vi "CFPI.vi"() -> ()   [LabVIEW 2014]
uses:
  <vilib>/Utility/file.llb/Write To Spreadsheet File (DBL).vi
panel:
  out "Elapsed time":dbl
  in  "Sin intervals":u32=40 caption="Sin" min=1 step=1
  in  "stop":bool
  in  "Matlab / Excel":bool
  in  "D intervals":u32=40 caption="D" min=1 step=1
  in  "Speed":u32=1 min=1 step=1
  in  "Scaled Time simulation":bool
  in  "Automatic D":bool caption="Automatic D values"
  in  "Write to file":bool
  in  "Initial conditions":bool
  in  "D_max":dbl=0.25 min=0.0 step=0.001 format="%#.5f"
  in  "D_min":dbl=0.01 min=0.0 step=0.001 format="%#.5f"
  in  "Do":dbl=40.0 caption="Sin_max" min=0.0
  in  "Od":dbl caption="Sin_min" min=0.0
  in  "czas pomiaru":dbl=400.0 caption="Measurement time"
  in  "czas stabilizacji":dbl=600.0 caption="Response formation time"
  out "D":dbl format="%.3f"
  out "X Chart":dbl(graph) caption="P Chart 2"
  out "P Chart":dbl(graph)
  in  "Tab Control":T1(tab)
  out "XY Graph 1":cluster{dbl[], dbl[]}[](graph)
  out "XY Graph 2":cluster{dbl[], dbl[]}[](graph)
  out "XY Graph 3":cluster{dbl[], dbl[]}[](graph)
  out "XY Graph 4":cluster{dbl[], dbl[]}[](graph)
  out "XY Graph 5":cluster{dbl[], dbl[]}[](graph)
  in  "tau":dbl=23.0 caption="delay"
  in  "S(0)":dbl
  in  "X(0)":dbl=1.0
  in  "P(0)":dbl
  in  "NIS":u32=10
  in  "Dt":dbl=0.1
  in  "Yp":dbl=3.68
  in  "Y":dbl=0.108
  in  "Ki":dbl=3.069
  in  "um":dbl=0.282 caption="m_m"
  in  "Ks":dbl=0.025
  in  "D5":dbl=0.25 caption="5" format="%#.5f"
  in  "D4":dbl=0.15 caption="4" format="%#.5f"
  in  "D3":dbl=0.1 caption="3" format="%#.5f"
  in  "D2":dbl=0.05 caption="2" format="%#.5f"
  in  "D1":dbl=0.01 caption="1" format="%#.5f"
  out "Sin":dbl format="%.3f"
  out "Substrate":dbl format="%.3f"
  out "Biomass":dbl format="%.3f"
  out "Product":dbl format="%.3f"
  out "Tank":cluster{dbl, dbl, dbl}(slide) scale=0.0..40.0
  # "Number of intervals"
  # "[s]"
  # "[h]"
  # "[h]"
  # "[g/L]"
  # "[g/L]"
  # "[1/h]"
  # "[1/h]"
  # "[1/h]"
  # "Parameters"
  # "Initial conditions"
  # "[1/h]"
  # "[g/L]"
  # "[g/L]"
  # "[g/L]"
  # "[g/L]"
  # "[g/L]"
  # "[g/g]"
  # "Simulation resolution"
  # "[g/g]"
  # "[h]"
  # "[h]"
  # "Manual D [1/h]"
  # "[g/L]"
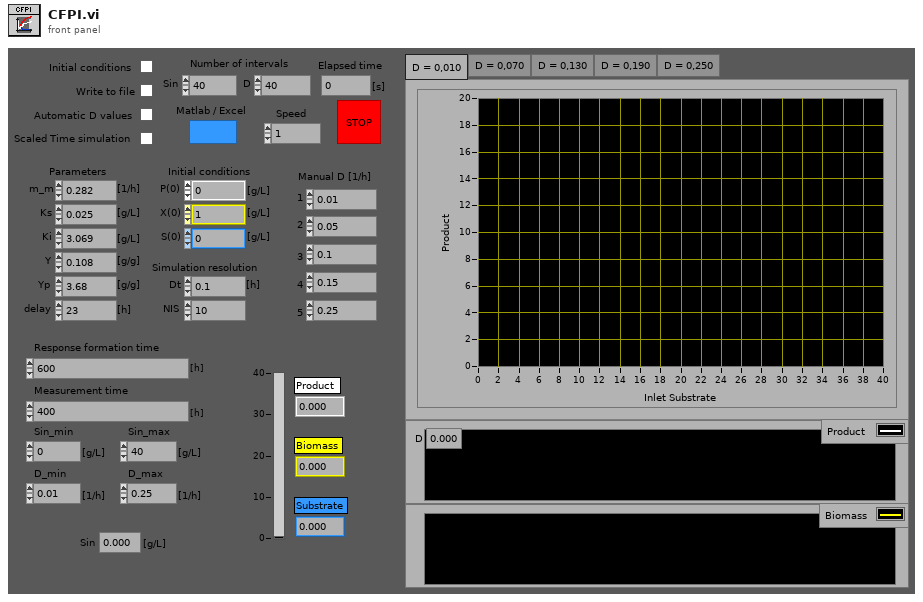
[diagram p1: front panel]
types:
  T1 = enum32{"Page 1", "Page 2", "Page 3", "Page 4", "Page 5"}
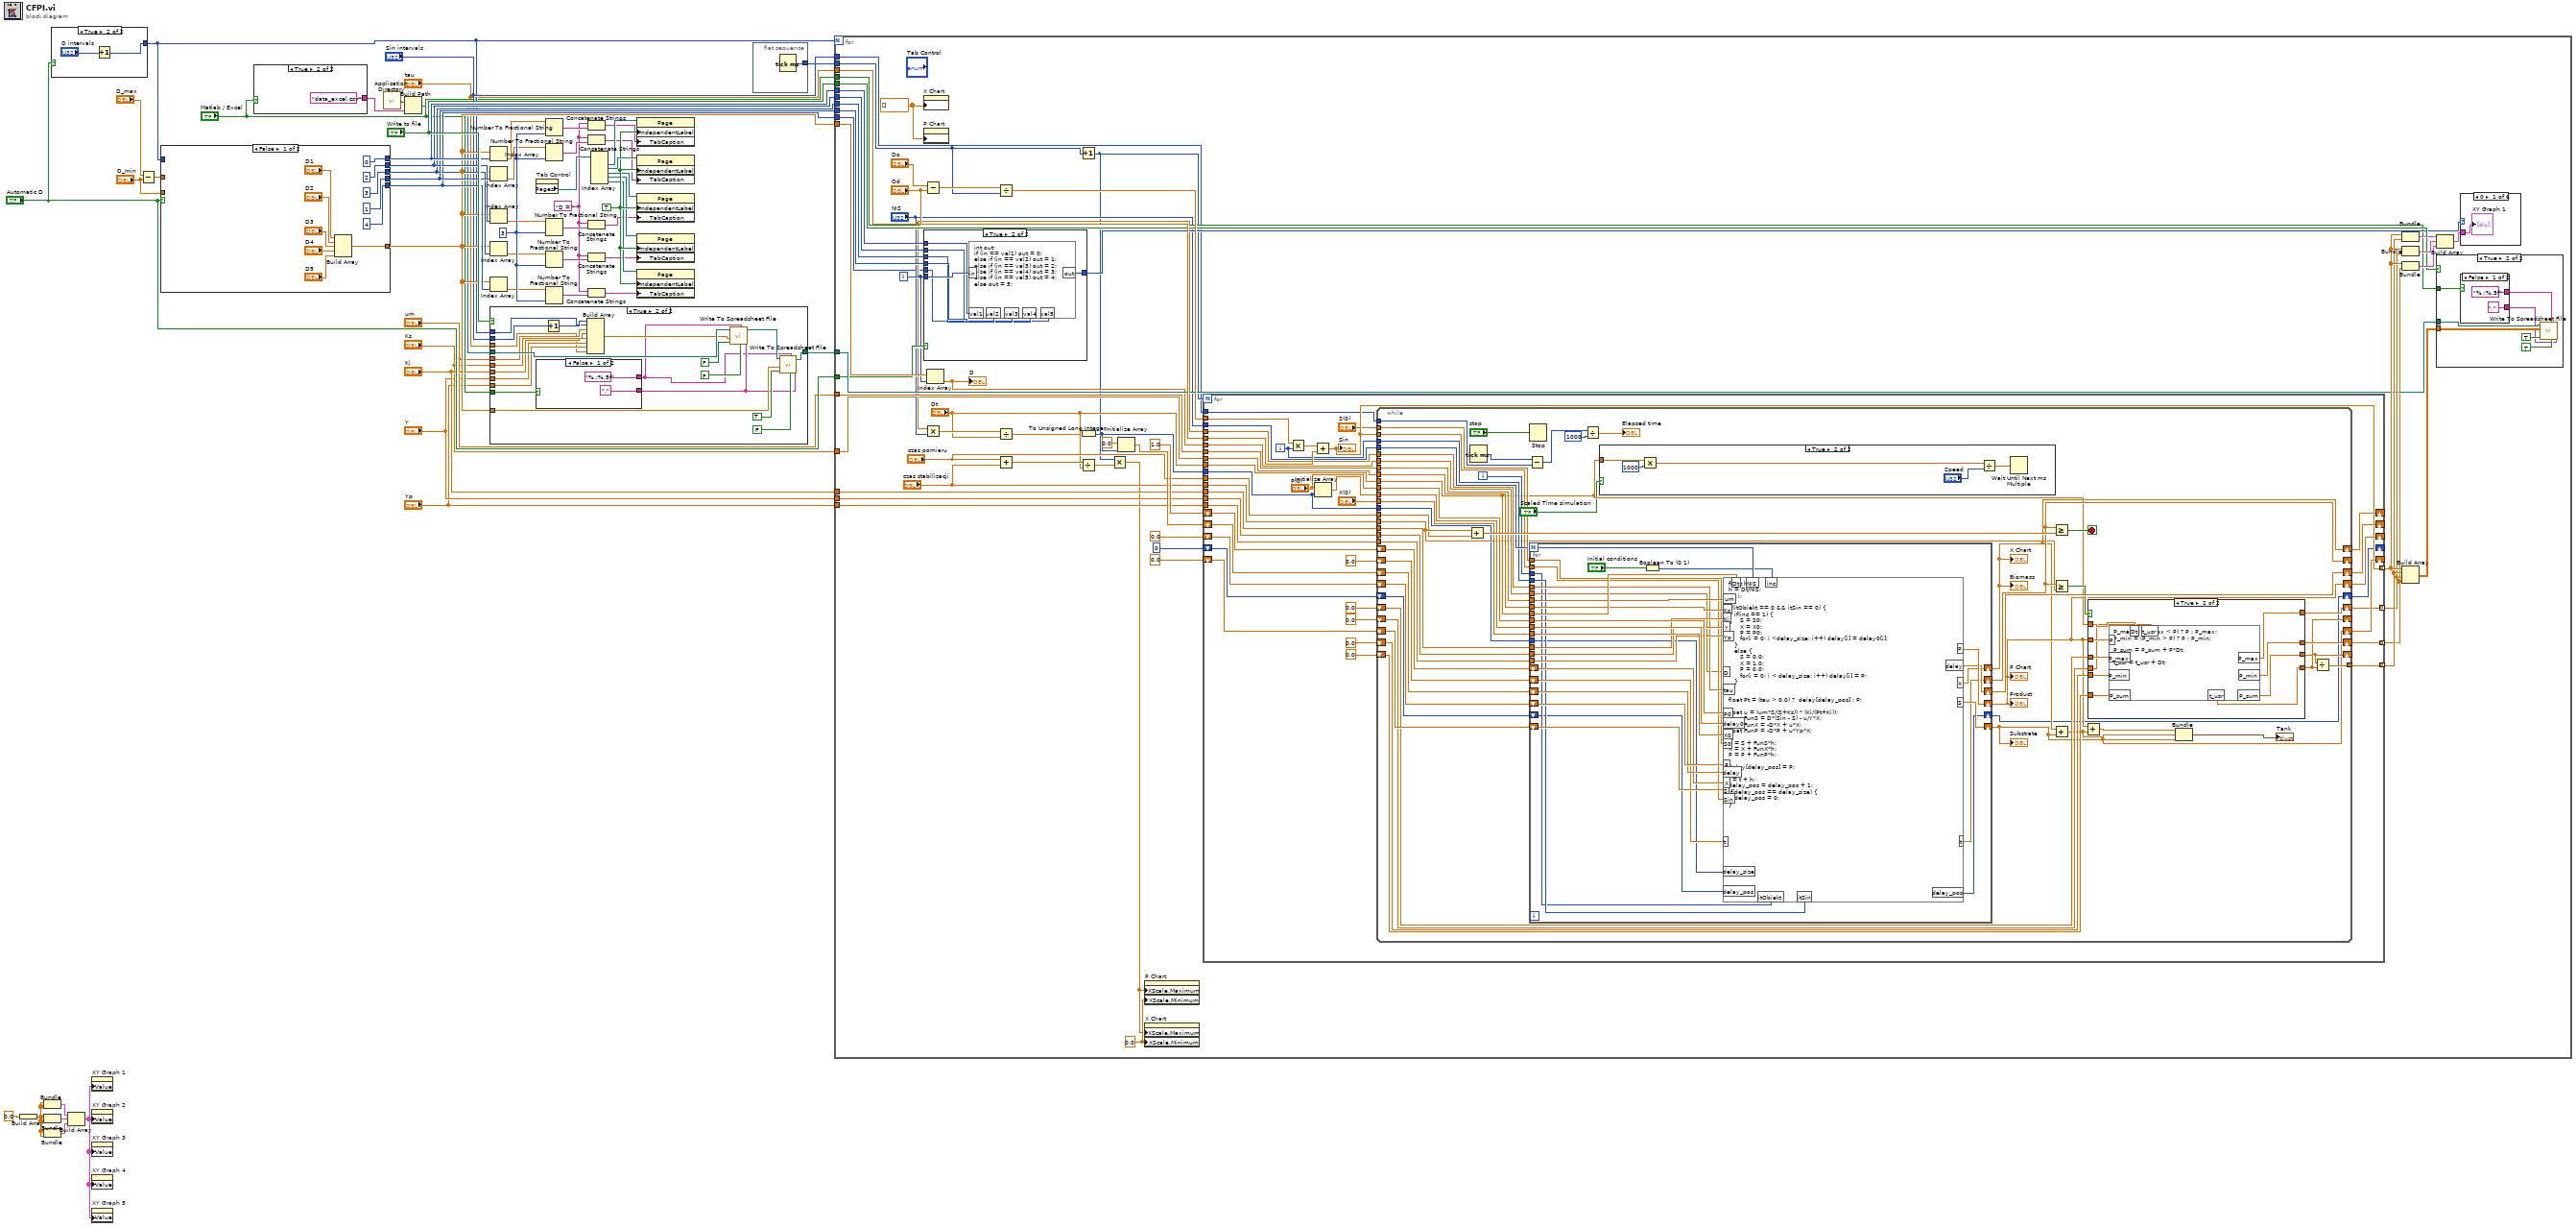
[diagram p0: block diagram]
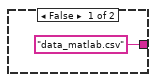
[diagram p2: hidden frame]
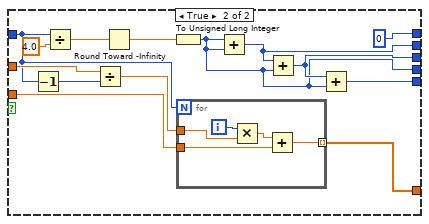
[diagram p3: hidden frame]
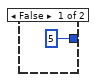
[diagram p4: hidden frame]
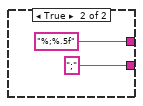
[diagram p6: hidden frame]
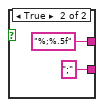
[diagram p9: hidden frame]
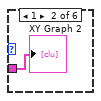
[diagram p10: hidden frame]
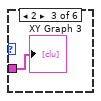
[diagram p11: hidden frame]
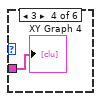
[diagram p12: hidden frame]
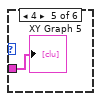
[diagram p13: hidden frame]
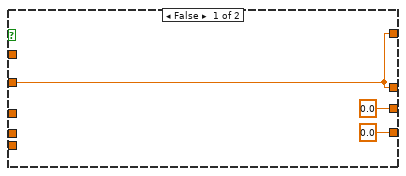
[diagram p15: hidden frame]
diagram:
  w41 = "D = "
  w48 = i16 3 ("precision (6)")
  w52 = TRUE ("Independent Label")
  n1 = Build Array(0.0) -> (w17:dbl[])
  n2 = Bundle(w17, w17) -> (w18:cluster{dbl[], dbl[]})  [unwired: 1 in]
  n3 = Bundle(w17, w17) -> (w19:cluster{dbl[], dbl[]})  [unwired: 1 in]
  n4 = Bundle(w17, w17) -> (w20:cluster{dbl[], dbl[]})  [unwired: 1 in]
  n5 = case shown="True" "Automatic D" {
    tunnel: [u32 5 w57] -> w21
    frame False {
    }
    frame True {
      n6 = Increment(x="D intervals") -> (x+1=w57:u32)
    }
  }
  n7 = Build Array(w18, w19, w20) -> (w15:cluster{dbl[], dbl[]}[])
  n8 = property on="XY Graph 1" class="XYGraph (strict)"("Value"=w15) -> ()  [unwired: 2 in, 2 out]
  n9 = property on="XY Graph 2" class="XYGraph (strict)"("Value"=w15) -> ()  [unwired: 2 in, 2 out]
  n10 = property on="XY Graph 3" class="XYGraph (strict)"("Value"=w15) -> ()  [unwired: 2 in, 2 out]
  n11 = property on="XY Graph 4" class="XYGraph (strict)"("Value"=w15) -> ()  [unwired: 2 in, 2 out]
  n12 = property on="XY Graph 5" class="XYGraph (strict)"("Value"=w15) -> ()  [unwired: 2 in, 2 out]
  n13 = Subtract(x="D_max", y="D_min") -> (x-y=w2:dbl)
  n14 = case shown="False" "Automatic D" {
    tunnel: [w64 w83] -> w23
    tunnel: w21 -> [_ w73]
    tunnel: w2 -> [_ w82]
    tunnel: [0 0] -> w28
    tunnel: [1 w71] -> w27
    tunnel: [2 w77] -> w26
    tunnel: [3 w76] -> w25
    tunnel: [4 w75] -> w24
    tunnel: "D_min" -> [_ w72]
    frame False {
      n15 = Build Array("D1", "D2", "D3", "D4", "D5") -> (w64:dbl[])
    }
    frame True {
      n16 = Decrement(x=w73) -> (x-1=w74:u32)
      n17 = Divide(x=w73, y=4.0) -> (x/y=w80:dbl)
      n18 = Divide(x=w82, y=w74) -> (x/y=w81:dbl)
      n19 = Round Toward -Infinity(1:w80) -> (0:w79:dbl)
      n20 = To Unsigned Long Integer(number=w79) -> (unsigned 32bit integer=w71:u32)
      n21 = for {
        N: w73 -> [_]
        tunnel: [w85] -> w83 mode=indexing
        tunnel: w81 -> [w87]
        tunnel: w72 -> [w84]
        i -> [w88]
        n22 = Multiply(x=w88, y=w87) -> (x*y=w86:dbl)
        n23 = Add(x=w86, y=w84) -> (x+y=w85:dbl)
      }
      n24 = Add(x=w71, y=w71) -> (x+y=w77:u32)
      n25 = Add(x=w77, y=w71) -> (x+y=w76:u32)
      n26 = Add(x=w76, y=w71) -> (x+y=w75:u32)
    }
  }
  n27 = case shown="True" "Matlab / Excel" {
    tunnel: ["data_matlab.csv" "data_excel.csv"] -> w11
    frame False {
    }
    frame True {
    }
  }
  n28 = call <vilib>:"Application Directory.vi"() -> ("Application Directory"=w13:path)
  n29 = Build Path(base path=w13, name or relative path=w11) -> (appended path=w10:path)
  n30 = Index Array(array=w23, index=w28) -> (element=w34:dbl)
  n31 = Index Array(array=w23, index=w27) -> (element=w33:dbl)
  n32 = Index Array(array=w23, index=w26) -> (element=w32:dbl)
  n33 = Index Array(array=w23, index=w25) -> (element=w31:dbl)
  n34 = Index Array(array=w23, index=w24) -> (element=w30:dbl)
  n35 = case shown="True" "Write to file" {
    tunnel: w10 -> [w91 w107]
    tunnel: [w91 w105] -> w36
    tunnel: w23 -> [_ w110]
    tunnel: w21 -> [_ w92]
    tunnel: "Sin intervals" -> [_ w93]
    tunnel: "Matlab / Excel" -> [_ w103]
    tunnel: "Ki" -> [_ w100]
    tunnel: "um" -> [_ w99]
    tunnel: "Ks" -> [_ w98]
    tunnel: "Y" -> [_ w97]
    tunnel: "Yp" -> [_ w96]
    tunnel: "tau" -> [_ w95]
    frame False {
    }
    frame True {
      n36 = case shown="False" w103 {
        tunnel: ["," ("delimiter (\\t)") ";" ("delimiter (\\t)")] -> w102
        tunnel: ["%.;%.5f" ("format (%.3f)") "%;%.5f" ("format (%.3f)")] -> w101
        frame False {
        }
        frame True {
        }
      }
      n37 = Increment(x=w93) -> (x+1=w94:u32)
      n38 = Build Array(w94, w92, w99, w98, w100, w97, w96, w95) -> (w106:dbl[])
      n39 = call-poly <vilib>:"Write To Spreadsheet File.vi"("delimiter (\\t)"=w102, "transpose? (no:F)"=FALSE, "format (%.3f)"=w101, "append to file? (new file:F)"=FALSE, "1D data"=w106, "file path (dialog if empty)"=w107) -> ("new file path (Not A Path if cancelled)"=w104:path)  [unwired: 2 in]
      n40 = call-poly <vilib>:"Write To Spreadsheet File.vi"("delimiter (\\t)"=w102, "transpose? (no:F)"=FALSE, "format (%.3f)"=w101, "append to file? (new file:F)"=TRUE, "1D data"=w110, "file path (dialog if empty)"=w104) -> ("new file path (Not A Path if cancelled)"=w105:path)  [unwired: 2 in]
    }
  }
  n41 = property on="Tab Control" class="TabCtl (strict)"() -> ("Pages"=w53:refnum<vi>[])  [unwired: 2 in, 2 out]
  n42 = Number To Fractional String(number=w34, precision (6)=w48) -> (F-format string=w43:string)  [unwired: 2 in]
  n43 = Number To Fractional String(number=w33, precision (6)=w48) -> (F-format string=w42:string)  [unwired: 2 in]
  n44 = Number To Fractional String(number=w32, precision (6)=w48) -> (F-format string=w44:string)  [unwired: 2 in]
  n45 = Number To Fractional String(number=w31, precision (6)=w48) -> (F-format string=w45:string)  [unwired: 2 in]
  n46 = Number To Fractional String(number=w30, precision (6)=w48) -> (F-format string=w46:string)  [unwired: 2 in]
  n47 = Concatenate Strings(w41, w43) -> (w38:string)
  n48 = Concatenate Strings(w41, w42) -> (w40:string)
  n49 = Concatenate Strings(w41, w44) -> (w39:string)
  n50 = Concatenate Strings(w41, w45) -> (w37:string)
  n51 = Concatenate Strings(w41, w46) -> (w47:string)
  n52 = Index Array(array=w53) -> (element #1=w55:refnum<vi>, element #2=w54:refnum<vi>, element #3=w51:refnum<vi>, element #4=w50:refnum<vi>, element #5=w49:refnum<vi>)  [unwired: 5 in]
  n53 = property class="Page"(reference=w55, "IndependentLabel"=w52, "TabCaption"=w38) -> ()  [unwired: 1 in, 2 out]
  n54 = property class="Page"(reference=w54, "IndependentLabel"=w52, "TabCaption"=w40) -> ()  [unwired: 1 in, 2 out]
  n55 = property class="Page"(reference=w51, "IndependentLabel"=w52, "TabCaption"=w39) -> ()  [unwired: 1 in, 2 out]
  n56 = property class="Page"(reference=w50, "IndependentLabel"=w52, "TabCaption"=w37) -> ()  [unwired: 1 in, 2 out]
  n57 = property class="Page"(reference=w49, "IndependentLabel"=w52, "TabCaption"=w47) -> ()  [unwired: 1 in, 2 out]
  n58 = flat-sequence {
    tunnel: [w117] -> w1
    frame #0 {
      n59 = Tick Count (ms)() -> (millisecond timer value=w117:u32)
    }
  }
  n60 = for {
    N: w21 -> [_]
    tunnel: "um" -> [w163]
    tunnel: "Write to file" -> [w146]
    tunnel: w36 -> [w148]
    tunnel: w23 -> [w145]
    tunnel: "Automatic D" -> [w144]
    tunnel: w28 -> [w141]
    tunnel: w27 -> [w140]
    tunnel: w26 -> [w139]
    tunnel: w25 -> [w138]
    tunnel: w24 -> [w119]
    tunnel: "Sin intervals" -> [w121]
    tunnel: "Matlab / Excel" -> [w135]
    tunnel: "Ki" -> [w133]
    tunnel: "tau" -> [w130]
    tunnel: "Ks" -> [w125]
    tunnel: "Y" -> [w124]
    tunnel: "Yp" -> [w123]
    tunnel: w1 -> [w118]
    i -> [w142]
    w147 = 0.0 ("X Scale.Range:Minimum")
    w137 = dbl[] [] ("History Data")
    n61 = property on="X Chart" class="WFChart (strict)"("History Data"=w137) -> ()  [unwired: 2 in, 2 out]
    n62 = property on="P Chart" class="WFChart (strict)"("History Data"=w137) -> ()  [unwired: 2 in, 2 out]
    n63 = case shown="True" w144 {
      tunnel: [w171 w177] -> w143
      tunnel: w142 -> [w171 w178]
      tunnel: w141 -> [_ w176]
      tunnel: w140 -> [_ w175]
      tunnel: w139 -> [_ w174]
      tunnel: w138 -> [_ w173]
      tunnel: w119 -> [_ w172]
      frame False {
      }
      frame True {
        n64 = formula code="int out;\nif (in == val1) out = 0;\nelse if (in == val2) out = 1;\nelse if (in == val3) out = 2;\nelse if (in == val4) out = 3;\nelse if (in == val5) out = 4;\nelse out = 5;"("in"=w178, "val1"=w176, "val2"=w175, "val3"=w174, "val4"=w173, "val5"=w172) -> ("out"=w177:i32)
      }
    }
    n65 = Subtract(x="Do", y="Od") -> (x-y=w165:dbl)
    n66 = Multiply(x=w130, y="NIS") -> (x*y=w132:dbl)
    n67 = Index Array(array=w145, index=w142) -> (element=w136:dbl)
    "D" <- w136
    n68 = Divide(x=w165, y=w121) -> (x/y=w164:dbl)
    n69 = Divide(x=w132, y="Dt") -> (x/y=w127:dbl)
    n70 = Add(x="czas pomiaru", y="czas stabilizacji") -> (x+y=w155:dbl)
    n71 = Increment(x=w121) -> (x+1=w120:u32)
    n72 = To Unsigned Long Integer(number=w127) -> (unsigned 32bit integer=w126:u32)
    n73 = Divide(x=w155, y="Dt") -> (x/y=w156:dbl)
    n74 = Multiply(x=w120, y=w156) -> (x*y=w122:dbl)
    n75 = Initialize Array(0.0 ("element"), w126) -> (w169:dbl[])
    n76 = property on="P Chart" class="WFChart (strict)"("XScale.Maximum"=w122, "XScale.Minimum"=w147) -> ()  [unwired: 2 in, 2 out]
    n77 = property on="X Chart" class="WFChart (strict)"("XScale.Maximum"=w122, "XScale.Minimum"=w147) -> ()  [unwired: 2 in, 2 out]
    n78 = for {
      N: w120 -> [_]
      shift-right: [w229] -> _
      shift-left: w169 -> [w231]
      shift-right: [w228] -> _
      shift-left: 0.0 ("P") -> [w221]
      shift-right: [w227] -> _
      shift-left: 1.0 ("X") -> [w225]
      shift-right: [w226] -> _
      shift-left: 0.0 ("S") -> [w224]
      tunnel: w164 -> [w220]
      tunnel: "Od" -> [w218]
      tunnel: w163 -> [w217]
      tunnel: w136 -> [w216]
      tunnel: [w215] -> w151 mode=indexing
      tunnel: [w214] -> w150 mode=indexing
      tunnel: [w207] -> w152 mode=indexing
      tunnel: [w212] -> w134 mode=indexing
      tunnel: "czas pomiaru" -> [w210]
      tunnel: "czas stabilizacji" -> [w209]
      tunnel: "Dt" -> [w208]
      tunnel: w133 -> [w204]
      tunnel: w130 -> [w203]
      tunnel: "NIS" -> [w202]
      tunnel: w126 -> [w199]
      shift-right: [w200] -> _
      shift-left: u32 0 ("delay_pos") -> [w201]
      tunnel: w125 -> [w198]
      tunnel: w124 -> [w197]
      tunnel: w123 -> [w196]
      tunnel: w118 -> [w195]
      i -> [w213]
      n79 = Multiply(x=w220, y=w213) -> (x*y=w219:dbl)
      n80 = Add(x=w219, y=w218) -> (x+y=w207:dbl)
      "Sin" <- w207
      n81 = Initialize Array("P(0)", w199) -> (w233:dbl[])
      n82 = while {
        tunnel: w208 -> [w254]
        shift-right: [w246] -> w228
        shift-left: w221 -> [w286]
        shift-right: [w245] -> w227
        shift-left: w225 -> [w285]
        shift-right: [w244] -> w226
        shift-left: w224 -> [w284]
        shift-right: [w287] -> w229
        shift-left: w231 -> [w283]
        shift-right: [w263] -> w214
        shift-left: 0.0 ("P_max") -> [w264]
        shift-right: [w279] -> w212
        shift-left: 0.0 ("P_min") -> [w262]
        shift-right: [w251] -> _
        shift-left: 0.0 ("P_sum") -> [w278]
        shift-right: [w256] -> _
        shift-left: 0.0 ("t_usr") -> [w277]
        tunnel: "P(0)" -> [w276]
        tunnel: w233 -> [w275]
        tunnel: "X(0)" -> [w274]
        tunnel: "S(0)" -> [w273]
        tunnel: w217 -> [w272]
        tunnel: w202 -> [w271]
        tunnel: w198 -> [w270]
        tunnel: w204 -> [w269]
        tunnel: w197 -> [w268]
        tunnel: w196 -> [w267]
        tunnel: w203 -> [w266]
        tunnel: [w265] -> w215
        tunnel: w207 -> [w261]
        tunnel: w216 -> [w260]
        tunnel: w213 -> [w257]
        shift-right: [w255] -> _
        shift-left: 0.0 ("t") -> [w259]
        tunnel: w209 -> [w253]
        tunnel: w210 -> [w252]
        tunnel: w199 -> [w243]
        shift-right: [w241] -> w200
        shift-left: w201 -> [w242]
        tunnel: w195 -> [w237]
        i -> [w258]
        stop <- w281 stop-if-true
        n83 = Add(x=w253, y=w252) -> (x+y=w282:dbl)
        n84 = Tick Count (ms)() -> (millisecond timer value=w236:u32)
        n85 = Subtract(x=w236, y=w237) -> (x-y=w239:u32)
        n86 = Stop(stop? (T)="stop") -> ()
        n87 = for {
          N: w271 -> [w336]
          shift-right: [w330] -> w287
          shift-left: w283 -> [w331]
          shift-right: [w335] -> w246
          shift-left: w286 -> [w333]
          shift-right: [w319] -> w245
          shift-left: w285 -> [w332]
          shift-right: [w334] -> w244
          shift-left: w284 -> [w317]
          tunnel: w254 -> [w329]
          tunnel: w258 -> [w309]
          tunnel: w276 -> [w328]
          tunnel: w275 -> [w327]
          tunnel: w274 -> [w326]
          tunnel: w273 -> [w318]
          tunnel: w272 -> [w325]
          tunnel: w270 -> [w324]
          tunnel: w269 -> [w323]
          tunnel: w268 -> [w322]
          tunnel: w267 -> [w321]
          tunnel: w266 -> [w320]
          tunnel: w261 -> [w316]
          tunnel: w260 -> [w312]
          shift-right: [w315] -> w255
          shift-left: w259 -> [w314]
          tunnel: w257 -> [w313]
          tunnel: w243 -> [w307]
          shift-right: [w306] -> w241
          shift-left: w242 -> [w308]
          n88 = Boolean To (0,1)(Boolean="Initial conditions") -> (0, 1=w310:i16)
          n89 = formula code="float h;\nh = Dt/NIS;\nint i;\n\nif(itObiekt == 0 && itSin == 0) {\n   if(inc == 1) {\n      S = S0;\n      X = X0;\n      P = P0;\n      for(i = 0; i <delay_size; i++) delay[i] = delay0[i];\n   }\n   else {\n      S = 0.0;\n      X = 1.0;\n      P = 0.0;\n      for(i = 0; i < delay_size; i++) delay[i] = P;\n   }\n}\n\nfloat Pt = (tau > 0.0) ?  delay[delay_pos] : P;\n\nfloat u = (um*S/(S+Ks)) * (Ki/(Pt+Ki));\nfloat FunS = D*(Sin - S) - u/Y*X;\nfloat FunX = -D*X + u*X;\nfloat FunP = -D*P + u*Yp*X;\n\nS = S + FunS*h;\nX = X + FunX*h;\nP = P + FunP*h;\n\ndelay[delay_pos] = P;\n\nt = t + h;\ndelay_pos = delay_pos + 1;\nif(delay_pos == delay_size) {\n   delay_pos = 0;\n}"("um"=w325, "S"=w317, "Ks"=w324, "Ki"=w323, "Sin"=w316, "D"=w312, "X"=w332, "Y"=w322, "Yp"=w321, "tau"=w320, "NIS"=w336, "Dt"=w329, "P"=w333, "P0"=w328, "X0"=w326, "S0"=w318, "delay"=w331, "itObiekt"=w309, "delay0"=w327, "t"=w314, "itSin"=w313, "inc"=w310, "delay_size"=w307, "delay_pos"=w308) -> ("P"=w335:dbl, "X"=w319:dbl, "S"=w334:dbl, "delay"=w330:dbl[], "t"=w315:dbl, "delay_pos"=w306:u32)
        }
        "P Chart" <- w246
        "X Chart" <- w245
        "Product" <- w246
        "Biomass" <- w245
        "Substrate" <- w244
        n90 = Divide(x=w239, y=u32 1000) -> (x/y=→"Elapsed time":dbl)
        n91 = case shown="True" "Scaled Time simulation" {
          tunnel: w254 -> [_ w302]
          frame False {
          }
          frame True {
            n92 = Multiply(x=w302, y=1000) -> (x*y=w303:dbl)
            n93 = Divide(x=w303, y="Speed") -> (x/y=w305:dbl)
            n94 = Wait Until Next ms Multiple(millisecond multiple=w305) -> ()  [unwired: 1 out]
          }
        }
        n95 = Greater Or Equal?(x=w255, y=w282) -> (x >= y?=w281:bool)
        n96 = Greater Or Equal?(x=w255, y=w253) -> (x >= y?=w280:bool)
        n97 = Add(x=w245, y=w244) -> (x+y=w248:dbl)
        n98 = Add(x=w246, y=w248) -> (x+y=w247:dbl)
        n99 = case shown="True" w280 {
          tunnel: [w288 w300] -> w263
          tunnel: [0.0 ("P_sum") w299] -> w251
          tunnel: [0.0 ("t") w298] -> w256
          tunnel: [w288 w297] -> w279
          tunnel: w246 -> [w288 w296]
          tunnel: w254 -> [_ w295]
          tunnel: w264 -> [_ w294]
          tunnel: w262 -> [_ w293]
          tunnel: w278 -> [_ w292]
          tunnel: w277 -> [_ w291]
          frame False {
          }
          frame True {
            n100 = formula code="P_max = (P_max < P) ? P : P_max;\nP_min = (P_min > P) ? P : P_min;\n\nP_sum = P_sum + P*Dt;\n\nt_usr = t_usr + Dt;"("P_max"=w294, "P_min"=w293, "P_sum"=w292, "P"=w296, "Dt"=w295, "t_usr"=w291) -> ("P_max"=w300:dbl, "P_min"=w297:dbl, "P_sum"=w299:dbl, "t_usr"=w298:dbl)
          }
        }
        n101 = Bundle(w247, w248, "S"=w244) -> (→"Tank":cluster{dbl, dbl, "S":dbl})  [unwired: 1 in]
        n102 = Divide(x=w251, y=w256) -> (x/y=w265:dbl)
      }
    }
    n103 = Bundle(w152, w151) -> (w159:cluster{dbl[], dbl[]})  [unwired: 1 in]
    n104 = Bundle(w152, w150) -> (w157:cluster{dbl[], dbl[]})  [unwired: 1 in]
    n105 = Bundle(w152, w134) -> (w158:cluster{dbl[], dbl[]})  [unwired: 1 in]
    n106 = Build Array(w152, w151, w150, w134) -> (w149:dbl[][])
    n107 = Build Array(w159, w157, w158) -> (w160:cluster{dbl[], dbl[]}[])
    n108 = case shown="True" w146 {
      tunnel: w149 -> [_ w183]
      tunnel: w148 -> [_ w182]
      tunnel: w135 -> [_ w181]
      frame False {
      }
      frame True {
        n109 = case shown="False" w181 {
          tunnel: ["," ("delimiter (\\t)") ";" ("delimiter (\\t)")] -> w180
          tunnel: ["%.;%.5f" ("format (%.3f)") "%;%.5f" ("format (%.3f)")] -> w179
          frame False {
          }
          frame True {
          }
        }
        n110 = call-poly <vilib>:"Write To Spreadsheet File.vi"("delimiter (\\t)"=w180, "transpose? (no:F)"=TRUE, "format (%.3f)"=w179, "append to file? (new file:F)"=TRUE, "2D data"=w183, "file path (dialog if empty)"=w182) -> ()  [unwired: 2 in, 1 out]
      }
    }
    n111 = case shown="0" w143 {
      tunnel: w160 -> [w190 w191 w192 w193 w194 _]
      frame 0 {
        "XY Graph 1" <- w190
      }
      frame 1 {
        "XY Graph 2" <- w191
      }
      frame 2 {
        "XY Graph 3" <- w192
      }
      frame 3 {
        "XY Graph 4" <- w193
      }
      frame 4 {
        "XY Graph 5" <- w194
      }
      frame 5, Default {
      }
    }
  }
